vi "get_vtemp.vi"(9 "COM":bool, 10 "VISA name":refnum<visa-resource-name>, 11 "cmd_std_header_t":T1) -> (2 "data out":u8[](array[numeric]), 3 "return":i32)   [LabVIEW 2016]
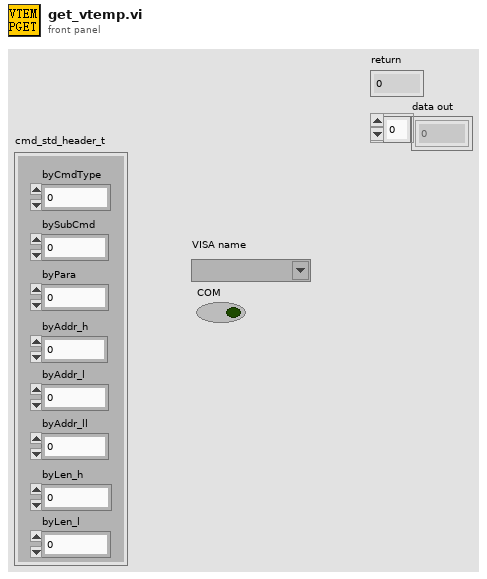
[diagram p1: front panel]
types:
  T1 = cluster{"byCmdType":u8, "bySubCmd":u8, "byPara":u8, "byAddr_h":u8, "byAddr_l":u8, "byAddr_ll":u8, "byLen_h":u8, "byLen_l":u8}
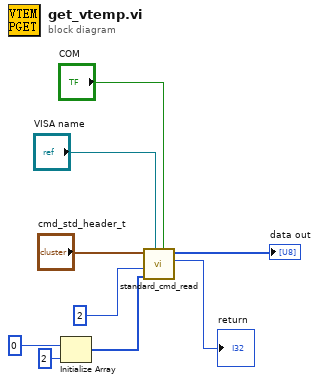
[diagram p0: block diagram]
diagram:
  n1 = Initialize Array(u8 0 ("element"), 2 ("dimension size")) -> (w4:u8[])
  n2 = call "standard_cmd_read.vi"("COM"="COM", "VISA name"="VISA name", "data"=w4, "dwLen"=u32 2, "cmd_std_header_t"="cmd_std_header_t") -> ("return"=→"return":i32, "data out"=→"data out":u8[])  [unwired: 5 in]
